vi "SetParametrAddress.vi"(8 "error in (no error)":errorcluster, 9 "Значение":dbl, 10 "Адрес параметра":u16 format="%04x", 11 "StepMotor in":refnum<class "StepMotor.lvclass">) -> (0 "error out":errorcluster, 3 "StepMotor out":refnum<class "StepMotor.lvclass">)   [LabVIEW 2010, in "StepMotor.lvclass"]
uses:
  StepMotor.lvclass
  StepMotor.lvclass/StepMotor.ctl
panel:
  in  "Адреса параметров":u16(ring) items=["0000", "0002", "0004", "0005", "0010", "0048", "0053", "0060", "0814", "0815", "0821", "0822", "0006", "0007", "0050", "0008", "0009", "000A", "000E", "0011", "0014", "000F", "0031", "0032", "0033", "0034", "0039", "0040", "0063", "0A16", "0A17", "0A18", "0A19", "0A1A", "0A1B", "0A1C", "081F", "0820", "000B", "000C", "000D", "0012", "0041", "0A12", "0A13", "0A14", "0A15", "081C", "0013", "001F", "0020", "0021", "0022", "0023", "0024", "0025", "0026", "0027", "0028", "0029", "002A", "002B", "002C", "0600", "0601", "0818", "0819", "081A", "0200", "0202", "0204", "0400", "040A", "0405", "040D", "0402", "0408", "0409", "0419", "040B", "040C", "0418", "040E", "0417", "0410", "040F", "0411", "0412", "0413", "0414", "0415", "0416", "0420", "0421", "0422", "0423", "0424", "0425", "0426", "0427", "0428", "0429", "042A", "042B", "042C", "0015", "0016", "001E", "0046", "0047", "0802", "0804", "0062", "0816", "0817", "0823", "0824", "0825", "0826", "0500", "0504", "0502", "0505", "0506", "0017", "0018", "001A", "001B", "001C", "001D", "0030", "0035", "0036", "0037", "0038", "0042", "0045", "0057", "0058", "0059", "0061", "0800", "0801", "081D", "081E", "0043", "0044", "0051", "0052", "0054", "0056", "081B", "0700", "0701", "0702", "0703", "0704", "0705", "0706", "0707", "0708", "0709", "070A", "070B", "070C", "070D", "070E", "070F", "0710", "0711", "0712", "0713", "0714", "0715", "0716", "0717", "0718", "0805", "0806", "0807", "0808", "0809", "080A", "080B", "080C", "080D", "080E", "080F", "0810", "0811", "0812", "070F", "0A01", "0A02", "0A03", "0A04", "0A05", "0A06", "0A07", "0A08", "0A09", "0A0A", "0A0B", "0A0C", "0A0D", "0A0E", "0A0F", "0A10", "0A11", "0A1D", "0A1E", ""]
  in  "Чтение запись":u16(ring) items=["0", "0", "0", "0", "0", "0", "0", "0", "0", "0", "0", "0", "0", "0", "0", "0", "0", "0", "0", "0", "0", "0", "0", "0", "0", "0", "0", "0", "0", "0", "0", "0", "0", "0", "0", "0", "0", "0", "0", "0", "0", "0", "0", "0", "0", "0", "0", "0", "0", "0", "0", "0", "0", "0", "0", "0", "0", "0", "0", "0", "0", "0", "0", "0", "0", "0", "0", "0", "0", "0", "0", "1", "0", "1", "0", "1", "1", "1", "1", "1", "1", "1", "1", "1", "1", "0", "1", "1", "1", "1", "1", "1", "0", "1", "1", "1", "1", "1", "0", "1", "1", "1", "1", "1", "1", "0", "0", "0", "0", "0", "0", "0", "0", "0", "0", "0", "0", "0", "1", "0", "0", "0", "0", "0", "0", "0", "0", "1", "0", "0", "0", "0", "0", "0", "1", "1", "0", "0", "0", "0", "0", "0", "0", "0", "0", "0", "0", "0", "0", "0", "0", "0", "0", "0", "0", "0", "0", "0", "0", "0", "0", "0", "0", "0", "0", "0", "0", "0", "1", "0", "0", "0", "0", "0", "0", "0", "0", "0", "0", "0", "0", "0", "0", "0", "0", "0", "0", "0", "0", "0", "0", "1", "0", "0", "0", "0", "0", "0", "0", "0", "0", "0", "0", "0", "0", "0", "0", "1", "1", "0", "0", ""]
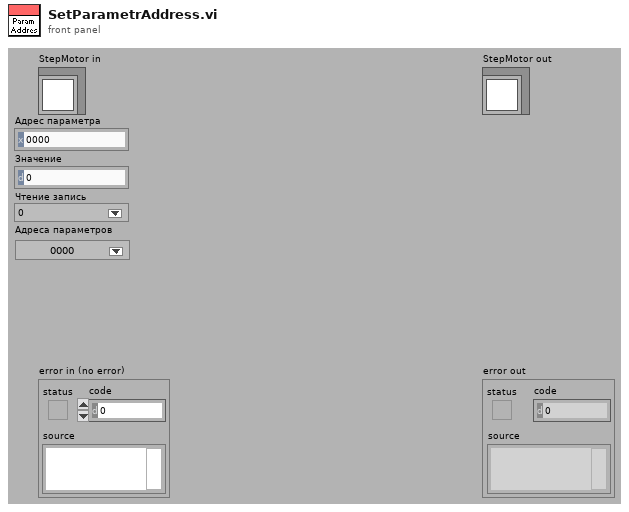
[diagram p1: front panel]
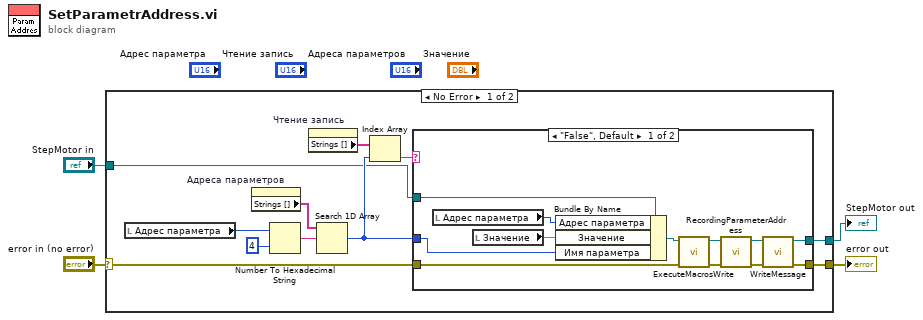
[diagram p0: block diagram]
diagram:
  n1 = case shown="No Error" "error in (no error)" {
    selector: "error in (no error)" -> [w8 w31]
    tunnel: [w9 w31] -> w3
    tunnel: [w10 w30] -> w1
    tunnel: "StepMotor in" -> [w6 w30]
    frame No Error {
      n2 = local read "Адрес параметра"() -> (w5:u16)
      n3 = property on="Адреса параметров" class="Ring (strict)"() -> ("Strings []"=w15:string[])  [unwired: 2 in, 2 out]
      n4 = Number To Hexadecimal String(1:i16 4 ("width (-)"), 2:w5) -> (0:w14:string)
      n5 = property on="Чтение запись" class="Ring (strict)"() -> ("Strings []"=w12:string[])  [unwired: 2 in, 2 out]
      n6 = Search 1D Array(1D array=w15, element=w14) -> (index of element=w7:i32)  [unwired: 1 in]
      n7 = Index Array(array=w12, index=w7) -> (element=w11:string)
      n8 = case shown="\"False\", Default" w11 {
        tunnel: [w17 w28] -> w10
        tunnel: [w16 w29] -> w9
        tunnel: w8 -> [w25 w29]
        tunnel: w7 -> [w23 _]
        tunnel: w6 -> [w22 w28]
        frame "False", Default {
          n9 = local read "Адрес параметра"() -> (w24:u16)
          n10 = local read "Значение"() -> (w20:dbl)
          n11 = Bundle By Name(cluster=w22, "Адрес параметра"=w24, "Значение"=w20, "Имя параметра"=w23) -> (w21:refnum<class "StepMotor.lvclass">)
          n12 = call-dynamic "ExecuteMacrosWrite.vi"("error in (no error)"=w25, "StepMotor in"=w21) -> ("error out"=w26:errorcluster, "StepMotor out"=w27:refnum<class "StepMotor.lvclass">)  [unwired: 8 in]
          n13 = call "RecordingParameterAddress.vi"("error in (no error)"=w26, "StepMotor in"=w27) -> ("error out"=w18:errorcluster, "StepMotor out"=w19:refnum<class "StepMotor.lvclass">)  [unwired: 8 in]
          n14 = call-dynamic "WriteMessage.vi"("error in (no error)"=w18, "StepMotor in"=w19) -> ("error out"=w16:errorcluster, "StepMotor out"=w17:refnum<class "StepMotor.lvclass">)  [unwired: 8 in]
        }
        frame "True" {
        }
      }
    }
    frame Error {
    }
  }
  "error out" <- w3
  "StepMotor out" <- w1
